vi "preciovscosto.vi"(8 "error in (no error)":errorcluster, 11 "UI Actor in":refnum<class "UI Actor.lvclass">) -> (0 "error out":errorcluster, 3 "UI Actor out":refnum<class "UI Actor.lvclass">)   [LabVIEW 2019, in "UI Actor.lvlib" / "UI Actor.lvclass"]
uses:
  UI Actor.lvclass
  UI Actor.lvclass/UI Actor.ctl
  <vilib>/ActorFramework/Message Enqueuer/Message Enqueuer.lvclass/Message Enqueuer.ctl
  Actor M Messages/Update M Msg/Update M Msg.lvclass/Update M Msg.ctl
  <vilib>/ActorFramework/Message Enqueuer/Enqueue.vi
  Soda Actor Messages/ActualizarTabla Msg/ActualizarTabla Msg.lvclass
  C:/Program Files (x86)/National Instruments/LabVIEW 2019/vi.lib/ActorFramework/Message/Message.lvclass
  Actor M Messages/Update M Msg/Update M Msg.lvclass
  <vilib>/ActorFramework/Message Priority Queue/Priority Enqueue.vi
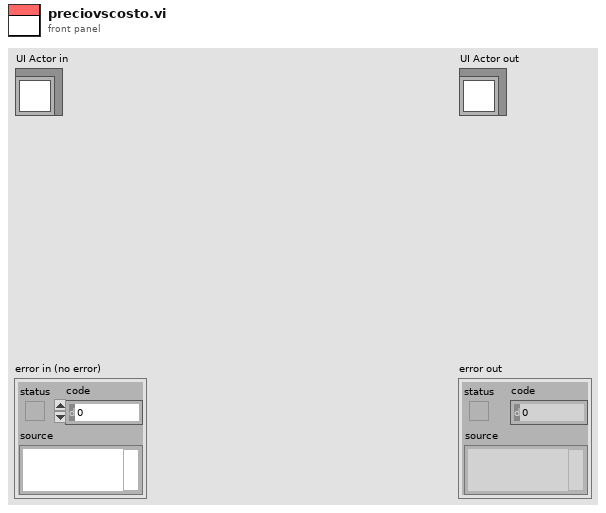
[diagram p1: front panel]
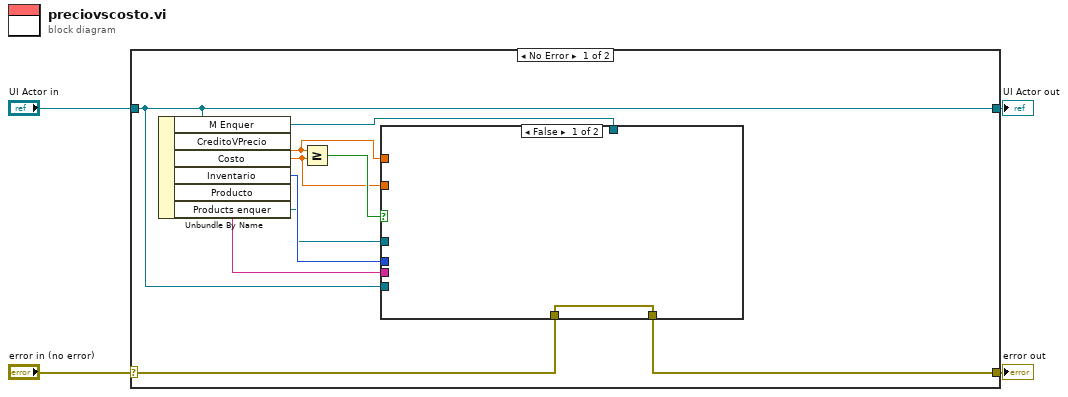
[diagram p0: block diagram]
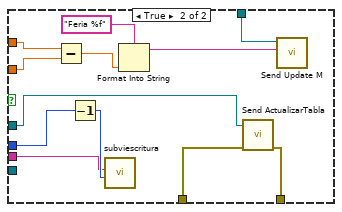
[diagram p2: hidden frame]
diagram:
  n1 = case shown="No Error" "error in (no error)" {
    selector: "error in (no error)" -> [w6 w29]
    tunnel: [w5 w29] -> w3
    tunnel: [w8 w28] -> w1
    tunnel: "UI Actor in" -> [w8 w28]
    frame No Error {
      n2 = Unbundle By Name(w8) -> ("M Enquer"=w9:refnum<class "Message Enqueuer.lvclass">, "CreditoVPrecio"=w12:dbl, "Costo"=w11:dbl, "Inventario"=w13:i32, "Producto"=w10:string, "Products enquer"=w7:refnum<class "Message Enqueuer.lvclass">)
      n3 = Greater Or Equal?(x=w12, y=w11) -> (x >= y?=w14:bool)
      n4 = case shown="False" w14 {
        tunnel: w13 -> [_ w27]
        tunnel: w12 -> [_ w26]
        tunnel: w11 -> [_ w25]
        tunnel: w8 -> [_ _]
        tunnel: w10 -> [_ w23]
        tunnel: w9 -> [_ w19]
        tunnel: w7 -> [_ w16]
        tunnel: w6 -> [w15 w18]
        tunnel: [w15 w17] -> w5
        frame False {
        }
        frame True {
          n5 = Subtract(x=w26, y=w25) -> (x-y=w22:dbl)
          n6 = Decrement(x=w27) -> (x-1=w24:i32)
          n7 = call "subviescritura.vi"("Numeric"=w24, "section"=w23) -> ()  [unwired: 10 in]
          n8 = Format Into String(format string="Feria %f", w22) -> (resulting string=w20:string)  [unwired: 2 in, 1 out]
          n9 = call "Send ActualizarTabla.vi"("error in (no error)"=w18, "Message Enqueuer"=w16) -> ("error out"=w17:errorcluster)  [unwired: 8 in, 1 out]
          n10 = call "Send Update M.vi"("Update M"=w20, "Message Enqueuer"=w19) -> ()  [unwired: 8 in, 2 out]
        }
      }
    }
    frame Error {
    }
  }
  "error out" <- w3
  "UI Actor out" <- w1
